vi "create_packet.vi"(0 "packet_id":u16, 1 "type":T1=enum."spi", 5 "packets_left":u16 format="%x", 7 "payload_size":u16=3, 9 "instruction":T2=173 items=["default"=0, "write"=173, "read"=237, "clear"=205], 11 "address":u8, 12 "data":u8) -> (8 "output cluster":T3 {"instruction" items=["default"=0, "write"=173, "read"=237, "clear"=205]; "data" format="%x"; "address" format="%x"})   [LabVIEW 2018]
uses:
  packet_t.ctl
  packet_type_t.ctl
  spi_instructions.ctl
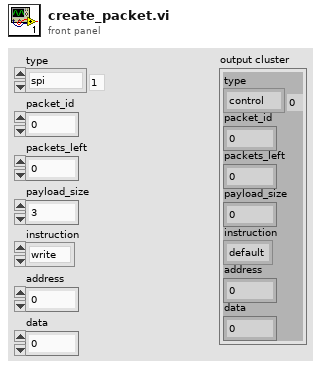
[diagram p1: front panel]
types:
  T1 = typedef "packet_type_t.ctl" = enum8{"control", "spi", "audio", "hdmi"}
  T2 = typedef "spi_instructions.ctl" = u8
  T3 = typedef "packet_t.ctl" = cluster{"type":T1, "packet_id":u16, "packets_left":u16, "payload_size":u16, "instruction":T2, "address":u8, "data":u8}
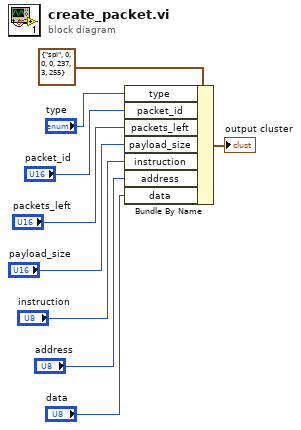
[diagram p0: block diagram]
diagram:
  n1 = Bundle By Name(cluster=T3 {"type"=enum."spi", "packet_id"=0, "packets_left"=0, "payload_size"=0, "instruction"=237, "address"=3, "data"=255} ("packet_t"), "type"="type", "packet_id"="packet_id", "packets_left"="packets_left", "payload_size"="payload_size", "instruction"="instruction", "address"="address", "data"="data") -> (→"output cluster":T3)
